vi "Transmit Dataset.vi"(8 "error in (no error)":errorcluster, 10 "Deliminator Char":string, 11 "OPC UA in":refnum<class "OPC UA.lvclass">) -> (0 "error out":errorcluster, 3 "OPC UA out":refnum<class "OPC UA.lvclass">)   [LabVIEW 2021, in "OPC UA.lvclass"]
uses:
  OPC UA.lvclass
  <vilib>/OPCUA/controls/Write Status.ctl
  OPC UA.lvclass/OPC UA.ctl
  <vilib>/OPCUA/controls/Write Variant Request.ctl
  <vilib>/OPCUA/controls/NodeId.ctl
  <vilib>/OPCUA/client/Multiple Write Variant.vi
  <vilib>/OPCUA/NI OPC UA Client.lvlib
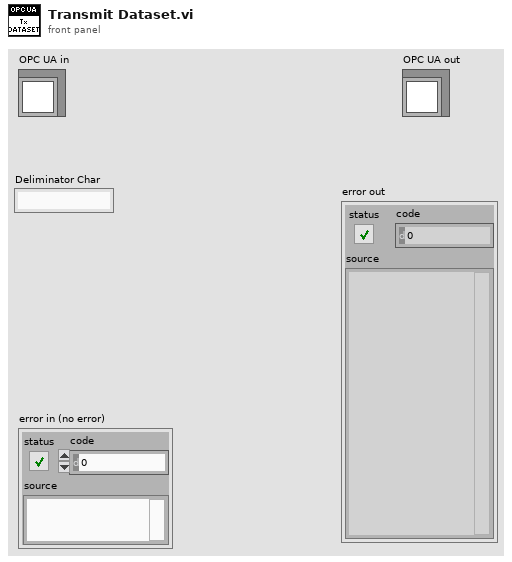
[diagram p1: front panel]
types:
  T1 = typedef "Write Status.ctl" = u32
  T2 = typedef "OPC UA Client Refnum.ctl" = refnum<k21>
  T3 = typedef "Write Variant Request.ctl" = cluster{"node ID":T4, "value":variant, "timestamp (current time)":timestamp, "node status":T1}
  T4 = typedef "NodeId.ctl" = string
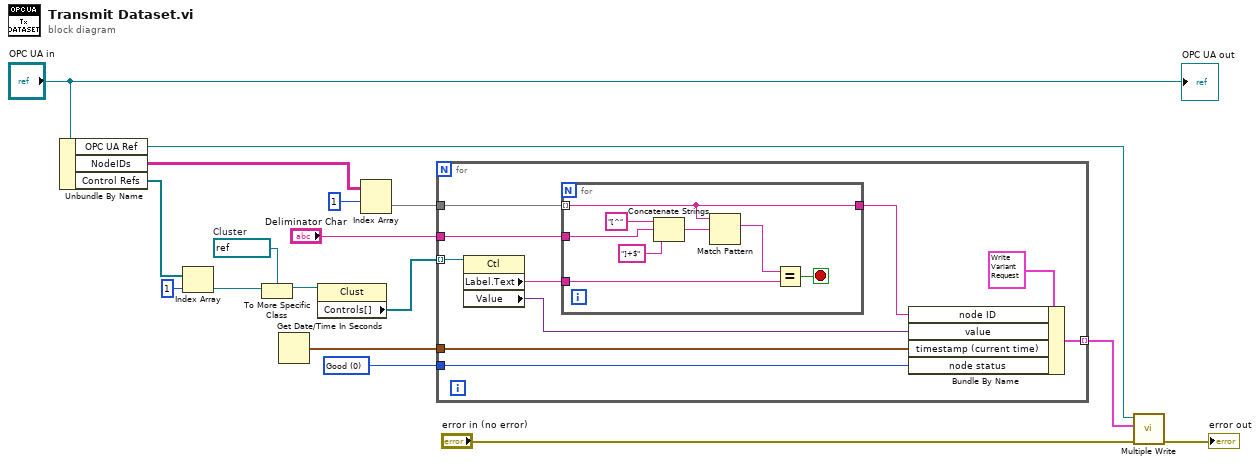
[diagram p0: block diagram]
diagram:
  w8 = refnum<vi> refnum  # Cluster
  w16 = T1 0 items=["Good"=0, "Uncertain"=1073741824, "Uncertain_InitialValue"=1083310080, "Uncertain_LastUsableValue"=1083179008, "Uncertain_SensorNotAccurate"=1083375616, "Uncertain_EngineeringUnitsExceeded"=1083441152, "Bad"=2147483648, "Bad_NoCommunication"=2150694912, "Bad_NotReadable"=2151284736, "Bad_NotWritable"=2151350272, "Bad_OutOfRange"=2151415808, "Bad_WaitingForInitialData"=2150760448] ("node status")
  n1 = Unbundle By Name("OPC UA in") -> ("OPC UA Ref"=w4:T2, "NodeIDs"=w13:string[][], "Control Refs"=w11:refnum<vi>[])
  n2 = Index Array(array=w11, index=1) -> (element=w9:refnum<vi>)
  n3 = To More Specific Class(target class=w8, reference=w9) -> (specific class reference=w7:refnum<vi>)  [unwired: 1 in, 1 out]
  n4 = Get Date/Time In Seconds() -> (seconds since 1Jan1904=w17:timestamp)
  n5 = property class="Clust"(reference=w7) -> ("Controls[]"=w6:refnum<vi>[])  [unwired: 1 in, 2 out]
  n6 = Index Array(array=w13, index (row)=1) -> (element=w12:string[])  [unwired: 1 in]
  n7 = for {
    tunnel: w6 -> [w27] mode=indexing
    tunnel: [w23] -> w5 mode=indexing
    tunnel: w17 -> [w22]
    tunnel: w12 -> [w25]
    tunnel: w16 -> [w20]
    tunnel: "Deliminator Char" -> [w18]
    n8 = property class="Ctl"(reference=w27) -> ("Label.Text"=w26:string, "Value"=w19:variant)  [unwired: 1 in, 2 out]
    n9 = for {
      tunnel: w26 -> [w35]
      tunnel: w25 -> [w30] mode=indexing
      tunnel: [w30] -> w21
      tunnel: w18 -> [w28]
      stop <- w34 stop-if-true
      n10 = Concatenate Strings("[^" ("string"), w28, "]+$" ("string")) -> (w33:string)
      n11 = Match Pattern(string=w30, regular expression=w33) -> (match substring=w29:string)  [unwired: 1 in, 3 out]
      n12 = Equal?(x=w29, y=w35) -> (x = y?=w34:bool)
    }
    n13 = Bundle By Name(cluster=T3 {"node ID"="", "value"=variant, "timestamp (current time)"=timestamp(0 s since 1904-01-01), "node status"=0} ("request"), "node ID"=w21, "value"=w19, "timestamp (current time)"=w22, "node status"=w20) -> (w23:T3)
  }
  n14 = call-poly <vilib>:"Multiple Write.vi"("error in (no error)"="error in (no error)", "requests"=w5, "OPC UA client refnum in"=w4) -> ("error out"=→"error out":errorcluster)  [unwired: 5 in, 3 out]
  "OPC UA out" <- "OPC UA in"
